vi "Lab6_QPSK1.vi"() -> ()   [LabVIEW 2019]
uses:
  <vilib>/addons/Modulation/Analog/support/mod_Set Error Source.vi
  <vilib>/addons/Modulation/Digital/Support/Common/Validators/mod_AWGN Validate.vi
  <vilib>/addons/Modulation/Digital/Impairments/subVIs/mod_createSeeds.vi
  <vilib>/addons/Modulation/Digital/Support/Common/Validators/mod_Validate Samples Per Symbol.vi
  <vilib>/addons/Modulation/Analog/support/Validators/mod_Validate Complex Waveform.vi
  <vilib>/addons/Modulation/Analog/support/Validators/mod_WFErrorHandler.vi
  <vilib>/addons/Modulation/Digital/Support/Common/Validators/mod_Generate Filter Coefficients Validate.vi
  <vilib>/addons/Modulation/Digital/General/subVIs/mod_Generate Filter Coefficients.vi
  <vilib>/addons/Modulation/Digital/General/MT Generate PSK System Parameters(M).vi
  <vilib>/addons/Modulation/Digital/General/subVIs/mod_Generate Bits PN Sequence.vi
  <vilib>/Analysis/1siggen.llb/Gaussian White Noise (obs 90).vi
  <vilib>/addons/Modulation/Digital/General/MT Generate PSK Synchronization Parameters (bit array).vi
  <vilib>/addons/Modulation/Digital/Demodulation/MT Calculate BER After Trigger (PN Sequence).vi
  <vilib>/addons/Modulation/Digital/General/MT Format Eye Diagram (complex).vi
  <vilib>/addons/Modulation/niDMT.lvlib
panel:
  in  "PSK type":u16(ring) items=["normal", "shifted", "offset"]
  in  "differential PSK":u16(ring) items=["disable", "enable"]
  out "Transmitted bitstream":i8[](array[numeric])
  out "Eye Diagram":cluster{"t0":dbl, "dt":dbl, "Y":dbl[]}[](graph)
  out "Constellation":T1(graph)
  out "BER":dbl format="%.4f"
  out "Receive bit stream":i8[](array[numeric])
  out "measurements":T2 {"phase offset (deg)" format="%.2f"; "frequency drift (Hz)" format="%.2f"; "frequency offset (Hz)" format="%.2f"}
  in  "Sync Location Uncertainly, Symbols":i32
  in  "Expecting Sync Location , Symbols":i32
  in  "Eb/N0 (10 dB)":dbl(knob)=10.0 scale=0.0..60.0
  in  "symbol rate (Hz)":dbl=1.0 format="%.2f"
  in  "I/Q (I)":enum16{"I", "Q"}(ring)
  in  "eye length":i32=1
  in  "Message":T3
  in  "M-PSK(4)":i32(ring) items=["2"=2, "4"=4, "8"=8, "16"=16]
  in  "Filter length(Symbols)":i32
  in  "Filter parameter":dbl format="%#_2p"
  in  "stop":bool
  in  "#Samples per symbol":i32(ring) items=["2"=2, "4"=4, "8"=8, "16"=16]
  in  "pulse shaping filter":u16(ring) items=["none", "Raised Cosine", "Root Raised Cos", "Gaussian"]
  # "DPSK and Offset-PSK"
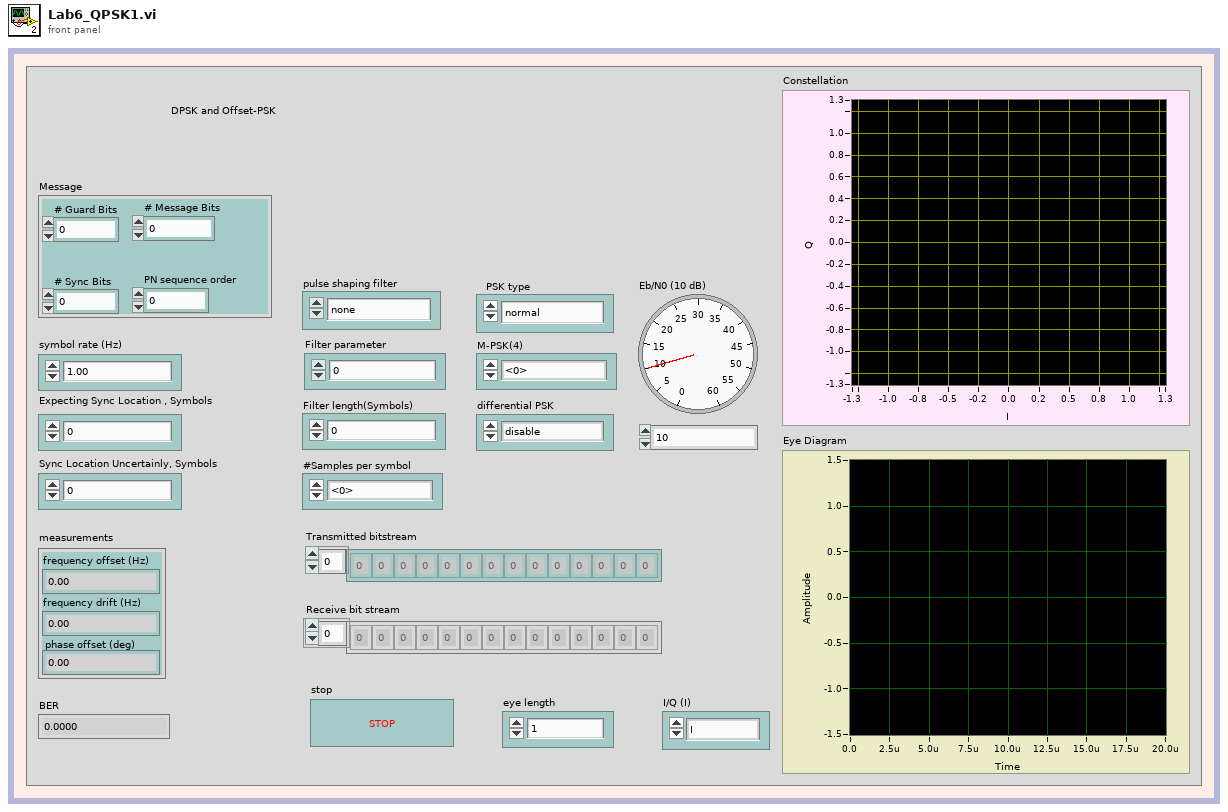
[diagram p1: front panel]
types:
  T1 = cluster{"Decimated Array":dbl[], "Decimated Array":dbl[]}[]
  T2 = cluster{"frequency offset (Hz)":dbl, "frequency drift (Hz)":dbl, "phase offset (deg)":dbl}
  T3 = cluster{"PN sequence order":i32, "# Guard Bits":i32, "# Sync Bits":i32, "# Message Bits":i32}
  T4 = cluster{"expected sync location (symbols)":i32, "sync sequence":cdb[], "sync location uncertainty (symbols)":i32, "sync indent (symbols)":i32}
  T5 = enum16{"FSK", "PSK", "QAM", "MSK", "PAM", "ASK", "CPM"}
  T6 = cluster{"samples per symbol (16)":i32, "symbol map":cdb[], "differential PSK":enum16{"disable", "enable"}, "PSK type":u16}
  T7 = typedef "niAMT.lvlib/Complex Data Waveform.ctl" = cluster{"t0":dbl, "dt":dbl, "Y":cdb[]}
  T8 = cluster{"constellation":dbl[], "oversampled data":dbl[]}[]
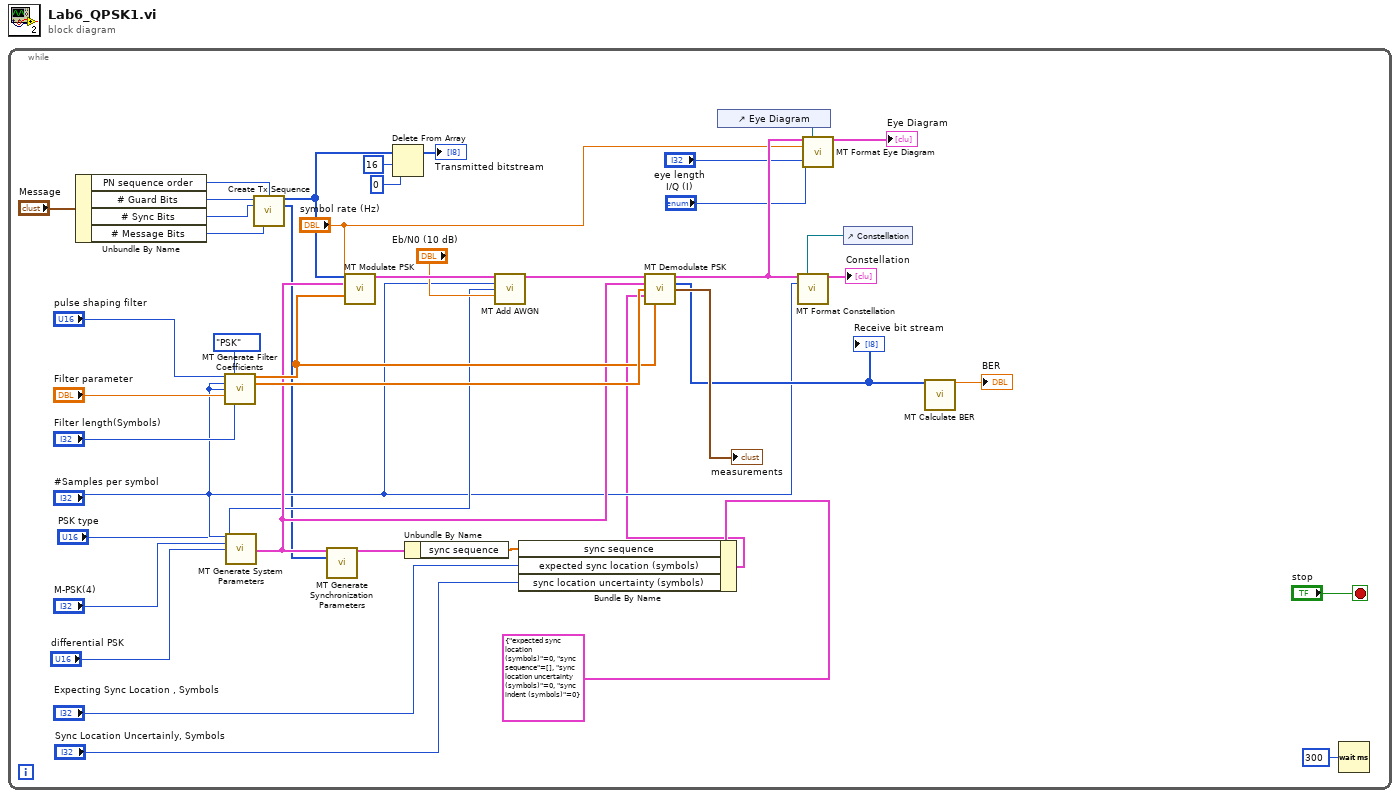
[diagram p0: block diagram]
diagram:
  n1 = while {
    stop <- "stop" stop-if-true
    n2 = Unbundle By Name("Message") -> ("PN sequence order"=w31:i32, "# Guard Bits"=w30:i32, "# Sync Bits"=w29:i32, "# Message Bits"=w28:i32)
    n3 = call <vilib>:"MT Generate Filter Coefficients.vi"("pulse shaping filter (none)"="pulse shaping filter", "modulation type"=T5."PSK", "pulse shaping samples per symbol (16)"="#Samples per symbol", "matched samples per symbol (16)"="#Samples per symbol", "filter parameter"="Filter parameter", "filter length (symbols)"="Filter length(Symbols)") -> ("pulse shaping filter coefficients"=w16:dbl[], "matched filter coefficients"=w17:dbl[])  [unwired: 7 in, 1 out]
    n4 = call-poly <vilib>:"MT Generate System Parameters.vi"("samples per symbol (16)"="#Samples per symbol", "PSK type"="PSK type", "M-PSK (4)"="M-PSK(4)", "differential PSK"="differential PSK") -> ("PSK system parameters"=w15:T6, "bits per symbol"=w14:i32)  [unwired: 9 in, 1 out]
    n5 = call "Create Tx Sequence.vi"("# Guard Bits (2)"=w30, "PN sequence order (9)"=w31, "# Sync Bits (20)"=w29, "# Message Bits"=w28) -> ("Output Bit Stream"=w27:i8[], "Last Sync Pattern"=w4:i8[])  [unwired: 8 in, 2 out]
    n6 = call-poly <vilib>:"MT Generate Synchronization Parameters.vi"("PSK system parameters"=w15, "sync bits"=w4) -> ("PSK synchronization parameters"=w26:T4)  [unwired: 12 in, 1 out]
    n7 = call <vilib>:"MT Modulate PSK.vi"("input bit stream"=w27, "PSK system parameters"=w15, "symbol rate (Hz)"="symbol rate (Hz)", "pulse shaping filter coefficients"=w16) -> ("output complex waveform"=w24:T7)  [unwired: 9 in, 2 out]
    n8 = Delete From Array(array=w27, length=16, index=0) -> (array with subset deleted=→"Transmitted bitstream":i8[])  [unwired: 1 out]
    n9 = Unbundle By Name(w26) -> ("sync sequence"=w9:cdb[])
    n10 = call <vilib>:"MT Add AWGN.vi"("input complex waveform"=w24, "samples per symbol (16)"="#Samples per symbol", "bits per symbol (1)"=w14, "Eb/N0 (10 dB)"="Eb/N0 (10 dB)") -> ("output complex waveform"=w23:T7)  [unwired: 9 in, 2 out]
    n11 = Bundle By Name(cluster=T4 {"expected sync location (symbols)"=0, "sync sequence"=[], "sync location uncertainty (symbols)"=0, "sync indent (symbols)"=0} ("synchronization parameters"), "sync sequence"=w9, "expected sync location (symbols)"="Expecting Sync Location , Symbols", "sync location uncertainty (symbols)"="Sync Location Uncertainly, Symbols") -> (w1:T4)
    n12 = call <vilib>:"MT Demodulate PSK.vi"("input complex waveform"=w23, "PSK system parameters"=w15, "matched filter coefficients"=w17, "synchronization parameters"=w1, "pulse shaping filter coefficients"=w16) -> ("recovered complex waveform"=w22:T7, "output bit stream"=w12:i8[], "measurements"=→"measurements":T2)  [unwired: 6 in, 2 out]
    "Receive bit stream" <- w12
    n13 = control-ref of="Eye Diagram"() -> (w40:refnum<vi>)
    n14 = call-poly <vilib>:"MT Format Eye Diagram.vi"("waveform"=w22, "eye diagram reference"=w40, "symbol rate (Hz)"="symbol rate (Hz)", "eye length"="eye length", "I/Q (I)"="I/Q (I)") -> ("eye diagram"=→"Eye Diagram":cluster{"t0":dbl, "dt":dbl, "Y":dbl[]}[])  [unwired: 2 in, 8 out]
    n15 = control-ref of="Constellation"() -> (w43:refnum<vi>)
    n16 = call <vilib>:"MT Format Constellation.vi"("waveform"=w22, "constellation reference"=w43, "samples per symbol"="#Samples per symbol") -> ("constellation graph"=→"Constellation":T8)  [unwired: 2 in, 10 out]
    n17 = call-poly <vilib>:"MT Calculate BER.vi"("input bit stream"=w12) -> ("BER"=→"BER":dbl)  [unwired: 10 in, 4 out]
    n18 = Wait (ms)(milliseconds to wait=u32 300) -> ()  [unwired: 1 out]
  }
